vi "WPI_RobotDriveArcadeDrive.vi"   [LabVIEW 2025]
doc: "Update motors by mapping joystick axes into motor values for arcade driving. Conventions, based on HID standard, are detailed on the mapping subVI panel, but are summarized as ...\ninput of -1 means forward and left, 0 means center, 1 means back or right.\n\noutput of -1 means motor power forward, 0 means no power, and 1 means reverse.\n\nThis software is licensed. Open the labview\\readme\\WPI Robotics Library Open Source License.txt file for more information."
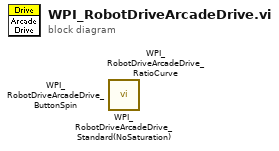
[diagram p0: block diagram]
diagram:
  n1 = call <vilib>:"WPI_RobotDriveArcadeDrive_Standard(NoSaturation).vi"() -> ()  [unwired: 9 in, 3 out]
  n2 = call <vilib>:"WPI_RobotDriveArcadeDrive_RatioCurve.vi"() -> ()  [unwired: 9 in, 3 out]
  n3 = call <vilib>:"WPI_RobotDriveArcadeDrive_ButtonSpin.vi"() -> ()  [unwired: 9 in, 3 out]
